vi "DoesScriptNumberExist.vi"(11 "Script Index":i32) -> (2 "file or folder exists?":bool)   [LabVIEW 2015]
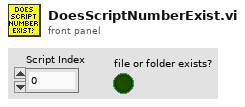
[diagram p1: front panel]
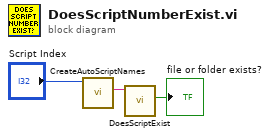
[diagram p0: block diagram]
diagram:
  n1 = call "CreateAutoScriptNames.vi"("Index"="Script Index") -> ("Concat String"=w2:string)  [unwired: 10 in]
  n2 = call "DoesScriptExist.vi"("File Name With Extension"=w2) -> ("file or folder exists?"=→"file or folder exists?":bool)  [unwired: 10 in]
